vi "Constants.vi"() -> ()   [LabVIEW 2015, in "Scriptable Model Interface Shared.lvlib"]
doc: "Use this Global VI to access the GUIDs assigned to the page resources of the Custom Device."
uses:
  Scriptable Model Interface Shared.lvlib
panel:
  in  "Tab Control":enum32{"GUIDS", "Constants", "Properties"}(tab)
  in  "5":string="f7ac7dab-51c1-4275-a848-02e1db423747"
  in  "4":string="82c4a5a8-7de7-4793-bb93-ff0d47a2e330"
  in  "3":string="cbaafd6c-859f-468b-83b0-c6fe6aff515c"
  in  "2":string="f384158c-1d49-4389-b57a-3875b0f073b3"
  in  "1":string="aa11a670-d93a-4470-97d1-1e78d67c0480"
  in  "Scriptable Model Interface":string="96f7262e-d258-407c-b907-d5b502be5bc3"
  in  "outputs section":string="output"
  in  "inputs section":string="input"
  in  "parameters json item property name":string="ScriptableModelInterfaceParameters"
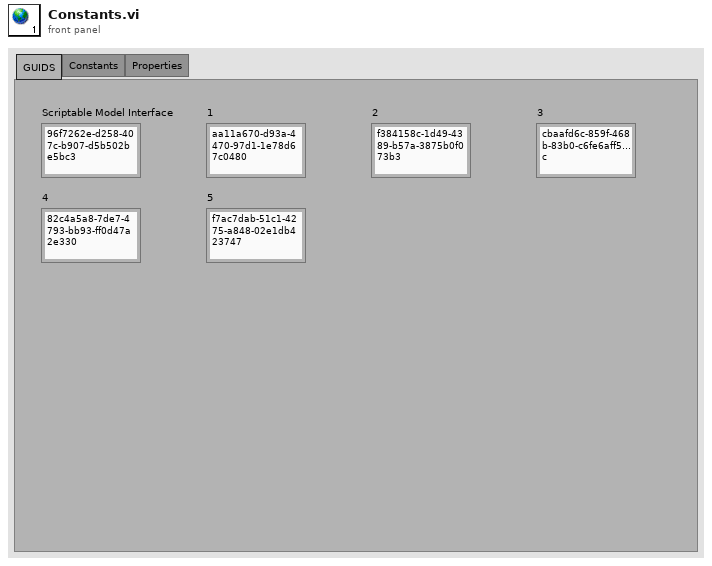
[diagram p1: front panel]
diagram:
